vi "inv_kin_test.vi"() -> ()   [LabVIEW 2011]
uses:
  <vilib>/Analysis/Matrix/Datatypes/RealMatrix.ctl
  <vilib>/Analysis/Matrix/NI_Matrix.lvlib
panel:
  out "RMS mismatch (mm/degree)":dbl
  out "number of function evaluations":i32
  out "Error":string
  out "f(minimum)":dbl
  out "Axis mismatch":dbl[](array[numeric])
  out "Axis positions out":dbl[](array[numeric])
  out "Pose":T1
  in  "Axis positions":dbl[](array[numeric])=[0.0, 0.0, 0.0, 0.0, 0.0, 0.0]
  # "Test inverse kinematics w.r.t. forward kinematics by starting with axis positions, converting to pose, then back again.  If there is gimbal lock, then there may be considerable mismatch in axis positions even though the pose is correct."
  # "RMS pose error (~microns)"
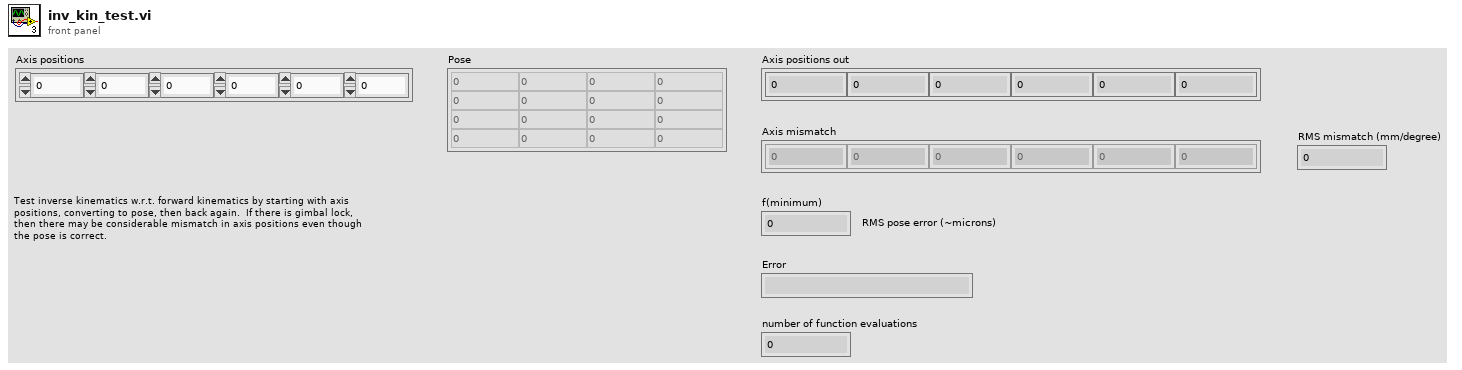
[diagram p1: front panel]
types:
  T1 = typedef "NI_Matrix.lvlib/RealMatrix.ctl" = dbl[][]
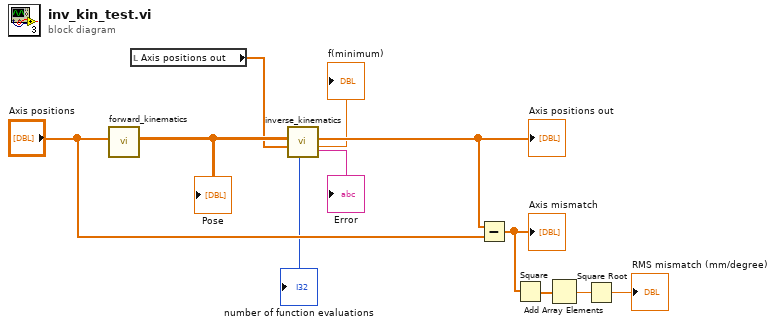
[diagram p0: block diagram]
diagram:
  n1 = call "forward_kinematics.vi"("Axis positions"="Axis positions") -> ("Pose"=w9:T1)  [unwired: 10 in]
  "Pose" <- w9
  n2 = local read "Axis positions out"() -> (w1:dbl[])
  n3 = call "inverse_kinematics.vi"("Initial axis positions"=w1, "Pose"=w9) -> ("f(minimum)"=→"f(minimum)":dbl, "Axis positions"=w11:dbl[], "Error"=→"Error":string, "number of function evaluations"=→"number of function evaluations":i32)  [unwired: 5 in, 1 out]
  "Axis positions out" <- w11
  n4 = Subtract(x=w11, y="Axis positions") -> (x-y=w3:dbl[])
  "Axis mismatch" <- w3
  n5 = Square(x=w3) -> (x^2=w4:dbl[])
  n6 = Add Array Elements(numeric array=w4) -> (sum=w5:dbl)
  n7 = Square Root(x=w5) -> (sqrt(x)=→"RMS mismatch (mm/degree)":dbl)
